vi "RC_receiver.vi"(2 "Scale":dbl=1.0 format="%#_13g", 3 "baud rate (9600)":u32=115200) -> ()   [LabVIEW 2017]
uses:
  <vilib>/myRIO/Instrument Drivers/Onboard IO/DIO/typedefs/DIO Reference.ctl
  <vilib>/myRIO/Common/Instrument Driver Framework/Utilities/typedefs/myRIO Generic Hardware Reference.ctl
  <vilib>/myRIO/Common/Instrument Driver Framework/Utilities/typedefs/Hardware Version Enum.ctl
  <vilib>/myRIO/Common/Instrument Driver Framework/Utilities/typedefs/myRIO v1.0 Reference.ctl
  <vilib>/myRIO/Common/Instrument Driver Framework/Utilities/typedefs/Generic FPGA Reference.ctl
  <vilib>/myRIO/Common/Instrument Driver Framework/myRIO v1.0/DIO/typedefs/DIO Channels List.ctl
  <vilib>/myRIO/Common/Instrument Driver Framework/myRIO v1.0/DIO/typedefs/DIO Channels Enum.ctl
  <vilib>/userdefined/High Color/nirio_resource_hc.ctl
  <vilib>/myRIO/Common/Instrument Driver Framework/Utilities/vis/Is FPGA Ref Available.vi
  <vilib>/myRIO/Common/Instrument Driver Framework/myRIO v1.0/DIO/vis/myRIO v1.1 Open DIO.vi
  <vilib>/myRIO/Instrument Drivers/Onboard IO/DIO/vis/Write.vi
  <vilib>/myRIO/Common/Instrument Driver Framework/Utilities/vis/Validate Channels.vi
  <vilib>/myRIO/Common/Instrument Driver Framework/myRIO v1.0/DIO/vis/myRIO v1.0 Reserve DIO.vi
  <vilib>/myRIO/Common/Instrument Driver Framework/myRIO v1.0/Resource Manager/vis/myRIO v1.0 Reserve Channel List.vi
  <vilib>/myRIO/Common/Instrument Driver Framework/myRIO v1.0/DIO/vis/myRIO v1.0 Build MUX Configuration DIO.vi
  <vilib>/myRIO/Common/Instrument Driver Framework/myRIO v1.0/Resource Manager/vis/myRIO v1.0 Reserve Channel.vi
  <vilib>/myRIO/Common/Instrument Driver Framework/myRIO v1.0/Resource Manager/vis/myRIO v1.0 Unreserve Channel.vi
  <vilib>/myRIO/Common/Instrument Driver Framework/myRIO v1.0/Resource Manager/vis/myRIO v1.0 Create Configuration List.vi
  <vilib>/myRIO/Common/Instrument Driver Framework/myRIO v1.0/Resource Manager/vis/myRIO v1.0 Build Mutex Name.vi
  <vilib>/Instr/_visa.llb/VISA Configure Serial Port (Instr).vi
  global.vi
  <vilib>/Utility/VariantDataType/GetNumericInfo.vi
  <vilib>/Utility/error.llb/Error Cluster From Error Code.vi
  <vilib>/myRIO/Common/Instrument Driver Framework/myRIO v1.0/myRIO v1.1 Open.vi
  <vilib>/myRIO/Common/Instrument Driver Framework/Utilities/vis/IO Manager.vi
  <vilib>/myRIO/Common/Instrument Driver Framework/Utilities/vis/Configuration Manager.vi
  <vilib>/myRIO/Common/Instrument Driver Framework/myRIO v1.0/Resource Manager/vis/myRIO v1.0 Configure IO.vi
  <vilib>/myRIO/Common/Instrument Driver Framework/myRIO v1.0/myRIO v1.0 Close.vi
  <vilib>/myRIO/Common/Instrument Driver Framework/myRIO v1.0/DIO/vis/myRIO v1.0 Write DIO.vi
  <vilib>/myRIO/Express VI/Onboard Devices/LED/LED Express VI.xnode
  <vilib>/myRIO/Instrument Drivers/Onboard IO/DIO/vis/myRIO DIO Open.xnode
  <vilib>/myRIO/Instrument Drivers/Onboard IO/DIO/DIO.lvlib
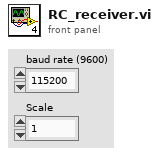
[diagram p1: front panel]
types:
  T1 = typedef "DIO.lvlib/DIO Reference.ctl" = cluster{"myRIO Reference":T2, "DIO Channels List":T6}
  T2 = typedef "myRIO Generic Hardware Reference.ctl" = cluster{"myRIO Model":T3, "myRIO Hardware Reference":T4}
  T3 = typedef "Hardware Version Enum.ctl" = enum16{"Unknown", "myRIO-1900", "myRIO-1950", "roboRIO", "NI ELVIS RIO CM"}
  T4 = typedef "myRIO v1.0 Reference.ctl" = cluster{"Generic FPGA Reference":T5, "Allow multiple opens":bool}
  T5 = typedef "Generic FPGA Reference.ctl" = refnum<k20>
  T6 = typedef "DIO Channels List.ctl" = T7[]
  T7 = typedef "DIO Channels Enum.ctl" = enum16{"Not Connected", "C/DIO0", "C/DIO1", "C/DIO2", "C/DIO3", "C/DIO4", "C/DIO5", "C/DIO6", "C/DIO7", "A/DIO0", "A/DIO1", "A/DIO2", "A/DIO3", "A/DIO4", "A/DIO5", "A/DIO6", "A/DIO7", "A/DIO8", "A/DIO9", "A/DIO10", "A/DIO11", "A/DIO12", "A/DIO13", "A/DIO14", "A/DIO15", "B/DIO0", "B/DIO1", "B/DIO2", "B/DIO3", "B/DIO4", "B/DIO5", "B/DIO6", "B/DIO7", "B/DIO8", "B/DIO9", "B/DIO10", "B/DIO11", "B/DIO12", "B/DIO13", "B/DIO14", "B/DIO15", "LED0", "LED1", "LED2", "LED3", "Button0", "DIO/DIO0", "DIO/DIO1", "DIO/DIO2", "DIO/DIO3", "DIO/DIO4", "DIO/DIO5", "DIO/DIO6", "DIO/DIO7", "DIO/DIO8", "DIO/DIO9", "SPI/CS0", "SPI/CS1", "SPI/CS2", "SPI/CS3", "LED RADIO (Green)", "LED RADIO (Red)", "LED COMM (Green)", "LED COMM (Red)", "LED MODE (Green)", "LED MODE (Red)"}
  T8 = typedef "nirio_resource_hc.ctl" = tag
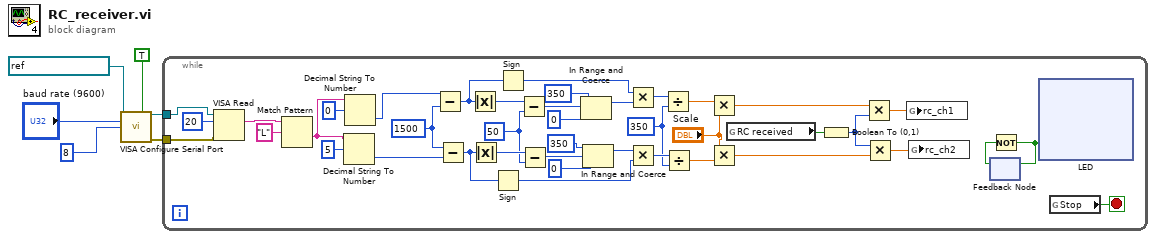
[diagram p0: block diagram]
diagram:
  n1 = call-poly "VISA Configure Serial Port"("VISA resource name"=refnum<visa-resource-name> "ASRL1::INSTR", "Enable Termination\nChar (T)"=TRUE ("Enable Termination\nChar (T)"), "baud rate (9600)"="baud rate (9600)", "data bits (8)"=u16 8) -> ("VISA resource name out"=w5:refnum<visa-resource-name>, "error out"=w6:errorcluster)  [unwired: 10 in]
  n2 = while {
    tunnel: w5 -> [w46]
    tunnel: w6 -> [w45]
    stop <- w44 stop-if-true
    w26 = 350 ("y")
    w30 = 50 ("y")
    w28 = 1500 ("y")
    n3 = VISA Read(VISA resource name=w46, byte count=u32 20 ("바이트 카운트"), error in (no error)=w45) -> (read buffer=w43:string)  [unwired: 3 out]
    n4 = Match Pattern(string=w43, regular expression="L" ("정규식")) -> (after substring=w40:string)  [unwired: 1 in, 3 out]
    n5 = Decimal String To Number(string=w40, offset=5 ("오프셋")) -> (number=w29:i32)  [unwired: 1 in, 1 out]
    n6 = Decimal String To Number(string=w40, offset=0 ("오프셋")) -> (number=w38:i32)  [unwired: 1 in, 1 out]
    n7 = Subtract(x=w38, y=w28) -> (x-y=w34:i32)
    n8 = Subtract(x=w28, y=w29) -> (x-y=w27:i32)
    n9 = Absolute Value(x=w34) -> (abs(x)=w37:i32)
    n10 = Absolute Value(x=w27) -> (abs(x)=w35:i32)
    n11 = Sign(1:w27) -> (0:w31:i32)
    n12 = Sign(1:w34) -> (0:w36:i32)
    n13 = Subtract(x=w37, y=w30) -> (x-y=w25:i32)
    n14 = Subtract(x=w35, y=w30) -> (x-y=w23:i32)
    n15 = In Range and Coerce(upper limit=350 ("상위 리미트"), x=w25, lower limit=0 ("하위 리미트")) -> (coerced(x)=w21:i32)  [unwired: 1 out]
    n16 = In Range and Coerce(upper limit=350 ("상위 리미트"), x=w23, lower limit=0 ("하위 리미트")) -> (coerced(x)=w22:i32)  [unwired: 1 out]
    n17 = Multiply(x=w36, y=w21) -> (x*y=w33:i32)
    n18 = Multiply(x=w22, y=w31) -> (x*y=w32:i32)
    n19 = Divide(x=w33, y=w26) -> (x/y=w16:dbl)
    n20 = Divide(x=w32, y=w26) -> (x/y=w17:dbl)
    n21 = Multiply(x=w16, y="Scale") -> (x*y=w11:dbl)
    n22 = Multiply(x="Scale", y=w17) -> (x*y=w8:dbl)
    n23 = global read "global.vi" "RC received"() -> (w10:bool)
    n24 = Boolean To (0,1)(Boolean=w10) -> (0, 1=w7:i16)
    n25 = Multiply(x=w11, y=w7) -> (x*y=w12:dbl)
    n26 = Multiply(x=w7, y=w8) -> (x*y=w9:dbl)
    n27 = global write "global.vi" "rc_ch1"(w12) -> ()
    n28 = global write "global.vi" "rc_ch2"(w9) -> ()
    n29 = feedback #1() -> (w14:bool)  [unwired: 1 in]
    n30 = Not(x=w14) -> (.not. x?=w13:bool)
    n31 = feedback-in #1(w13) -> ()
    n32 = xnode "LED"("LED0"=w13) -> ()  [unwired: 1 in, 1 out]
    n33 = global read "global.vi" "Stop"() -> (w44:bool)
  }
